vi "User Event Close.vi"(10 "Event Registration Refnum":refnum<event-registration>, 11 "user events":T1) -> (0 "error out":errorcluster)   [LabVIEW 2021, in "TSC Button Editor.lvclass"]
doc: "close all user events\n\n<b>Code Developed By:</b>\nTechnology Service Corporation\n1983 S Liberty Drive\nBloomington, IN 47403\nwww.tsc.com/atcs\n\nDeveloper:\nDaniel Coons"
uses:
  project/_button-editor/TSC Button Editor.lvclass
  project/_button-editor/User Events.ctl
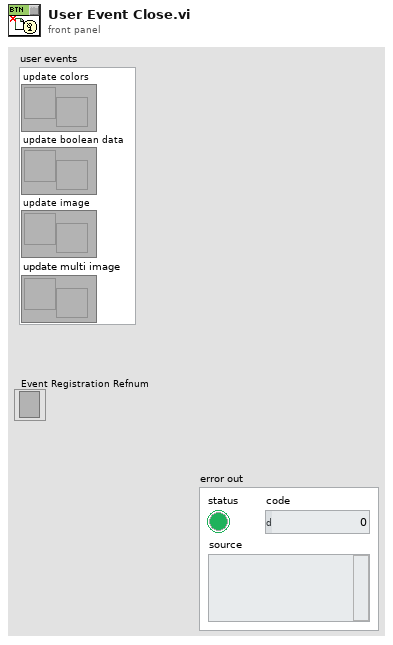
[diagram p1: front panel]
types:
  T1 = typedef "TSC Button Editor.lvclass/User Events.ctl" = cluster{"update colors":refnum<user-event>, "update boolean data":refnum<user-event>, "update image":refnum<user-event>, "update multi image":refnum<user-event>}
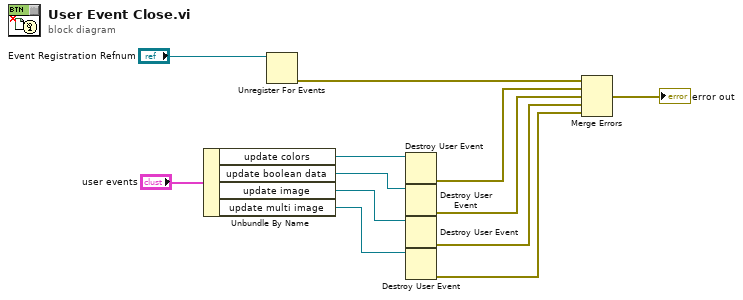
[diagram p0: block diagram]
diagram:
  n1 = Unbundle By Name("user events") -> ("update colors"=w10:refnum<user-event>, "update boolean data"=w9:refnum<user-event>, "update image"=w4:refnum<user-event>, "update multi image"=w3:refnum<user-event>)
  n2 = Unregister For Events(event registration refnum="Event Registration Refnum") -> (error out=w8:errorcluster)  [unwired: 1 in]
  n3 = Destroy User Event(user event=w10) -> (error out=w7:errorcluster)  [unwired: 1 in]
  n4 = Destroy User Event(user event=w9) -> (error out=w6:errorcluster)  [unwired: 1 in]
  n5 = Destroy User Event(user event=w4) -> (error out=w1:errorcluster)  [unwired: 1 in]
  n6 = Destroy User Event(user event=w3) -> (error out=w2:errorcluster)  [unwired: 1 in]
  n7 = Merge Errors(w8, w7, w6, w1, w2) -> (→"error out":errorcluster)
